vi "Write_Data.vi"(6 "Queues":T8, 8 "Status/Errors in":refnum<vi>, 9 "# Events to store":i32, 10 "Write data parameters in":T1 caption="Data Storage" {"Data storage"."Detector number" format="%#.0f"}) -> (0 "Status/Errors out":refnum<vi>, 2 "Write data parameters out":T1 {"Data storage"."Detector number" format="%#.0f"})   [LabVIEW 2013]
uses:
  Controls/Write_Data_Parameters.ctl
  Controls/Stop_Loop.ctl
  Controls/Data_Storage.ctl
  Controls/DB_Connection.ctl
  database/Connection.llb/Conn ObjectReference.ctl
  Controls/Data_Storage_Condition.ctl
  Controls/GPS_Timestamp.ctl
  Controls/Queues.ctl
  Controls/One_Second.ctl
  Controls/Get_Set_Statistics_Options2.ctl
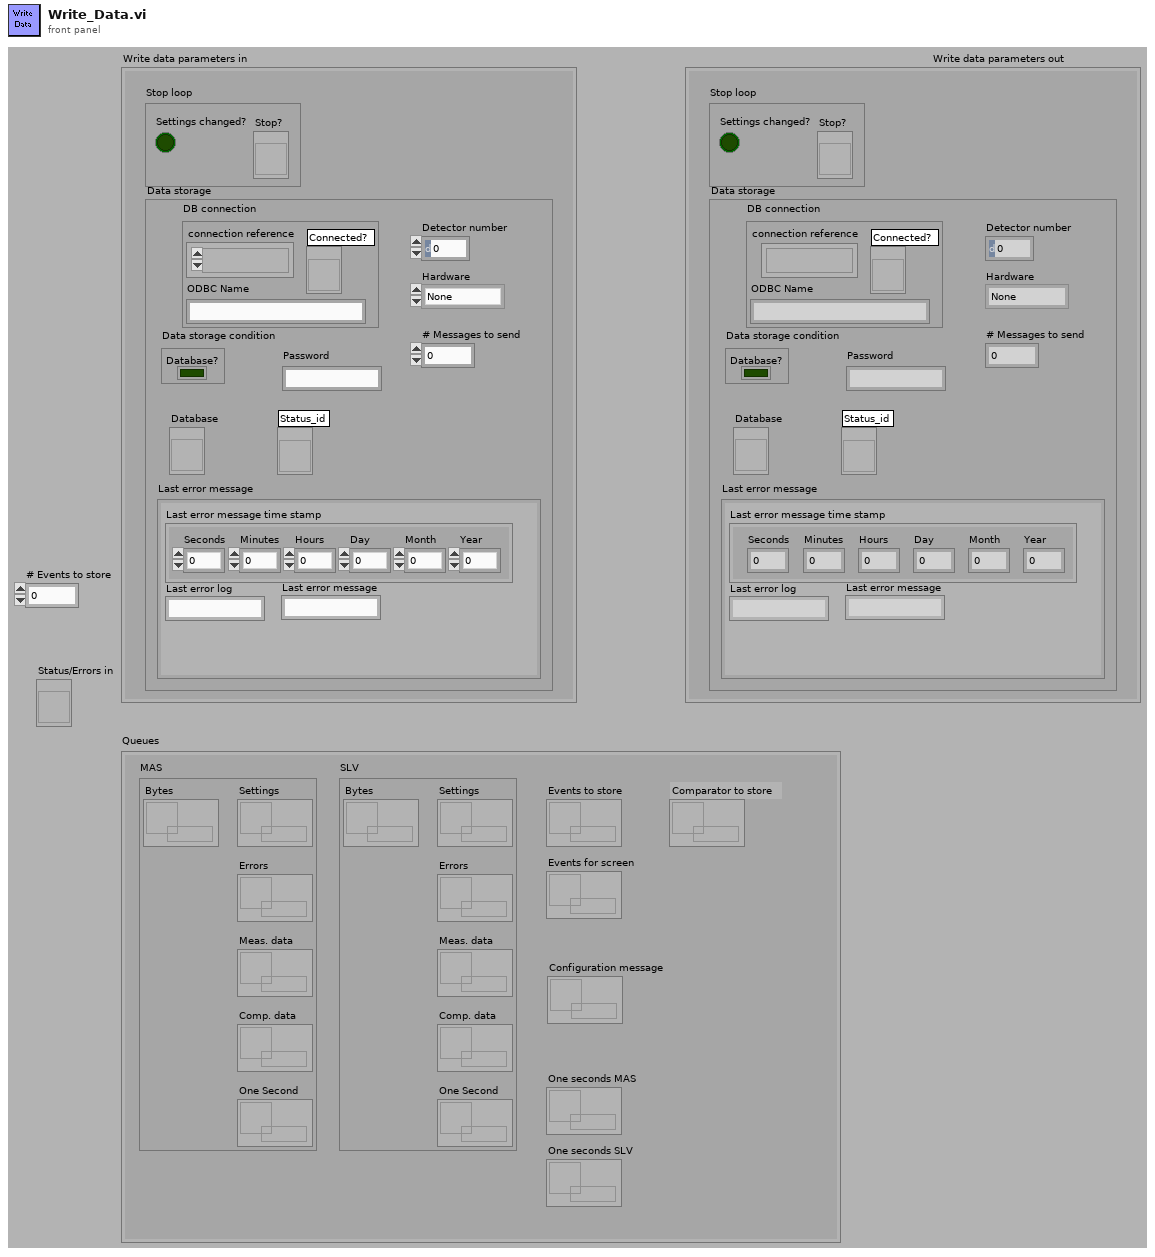
[diagram p1: front panel]
types:
  T1 = typedef "Write_Data_Parameters.ctl" = cluster{"Stop loop":T2, "Data storage":T3}
  T2 = typedef "Stop_Loop.ctl" = cluster{"Settings changed?":bool, "Stop?":refnum<vi>}
  T3 = typedef "Data_Storage.ctl" = cluster{"DB connection":T4, "Data storage condition":T6, "Detector number":u16, "# Messages to send":i32, "Database":refnum<vi>, "Password":string, "Last error message":cluster{"Last error message time stamp":T7, "Last error log":string, "Last error message":string}, "Status_id":refnum<vi>, "Hardware":enum8{"None", "HiSPARC I", "HiSPARC II", "HiSPARC III", "Unknown"}}
  T4 = typedef "DB_Connection.ctl" = cluster{"connection reference":T5, "Connected?":refnum<vi>, "ODBC Name":string}
  T5 = typedef "Conn ObjectReference.ctl" = refnum<k1>
  T6 = typedef "Data_Storage_Condition.ctl" = cluster{"Database?":bool}
  T7 = typedef "GPS_Timestamp.ctl" = cluster{"Seconds":u8, "Minutes":u8, "Hours":u8, "Day":u8, "Month":u8, "Year":u16}
  T8 = typedef "Queues.ctl" = cluster{"MAS":cluster{"Bytes":refnum<queue>, "Settings":refnum<queue>, "Errors":refnum<queue>, "Meas. data":refnum<queue>, "One Second":refnum<queue>, "Comp. data":refnum<queue>}, "SLV":cluster{"Bytes":refnum<queue>, "Settings":refnum<queue>, "Errors":refnum<queue>, "Meas. data":refnum<queue>, "One Second":refnum<queue>, "Comp. data":refnum<queue>}, "Events to store":refnum<queue>, "Events for screen":refnum<queue>, "One seconds MAS":refnum<queue>, "One seconds SLV":refnum<queue>, "Configuration message":refnum<queue>, "Comparator to store":refnum<queue>}
  T9 = typedef "Get_Set_Statistics_Options2.ctl" = enum16{"Get", "Set"}
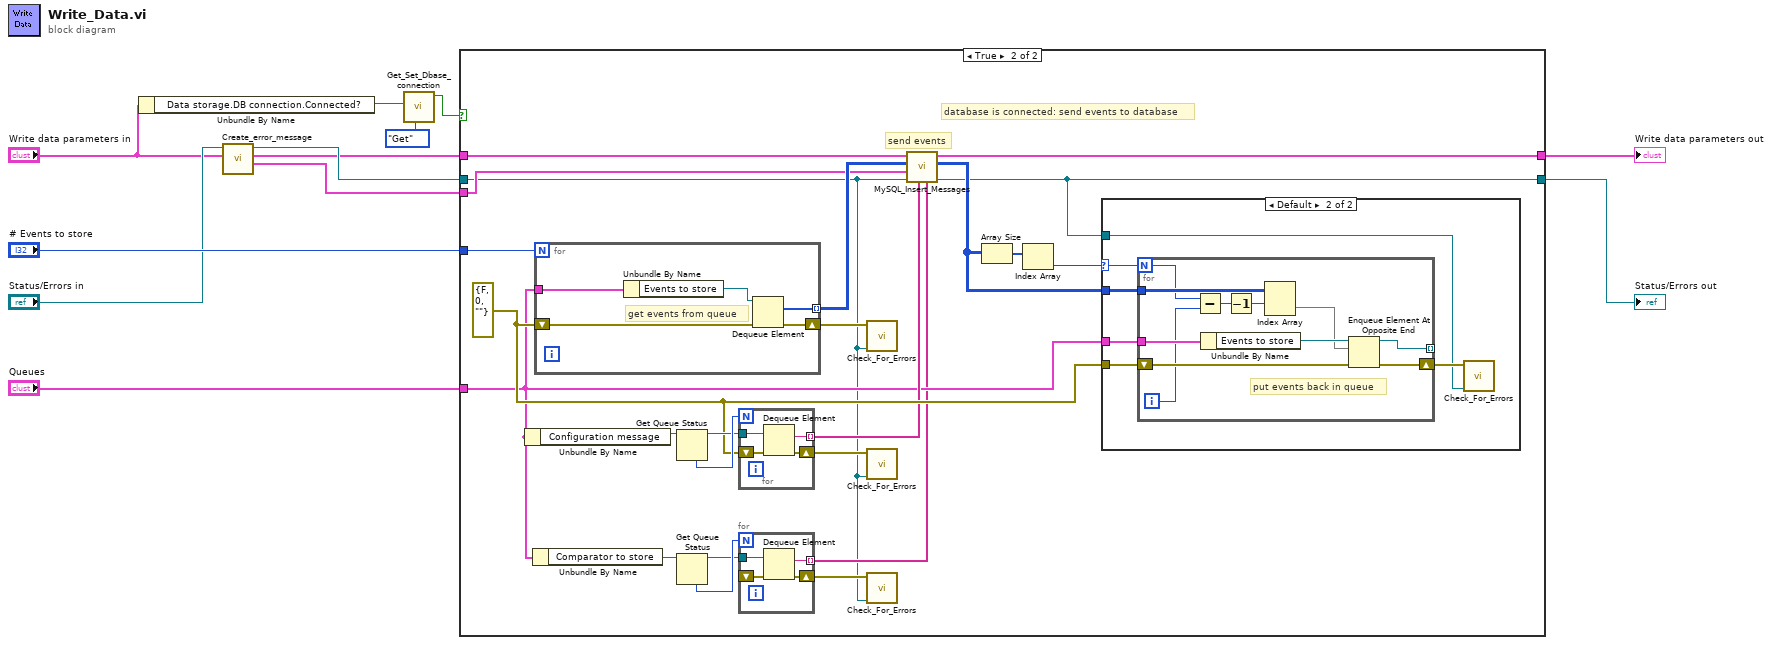
[diagram p0: block diagram]
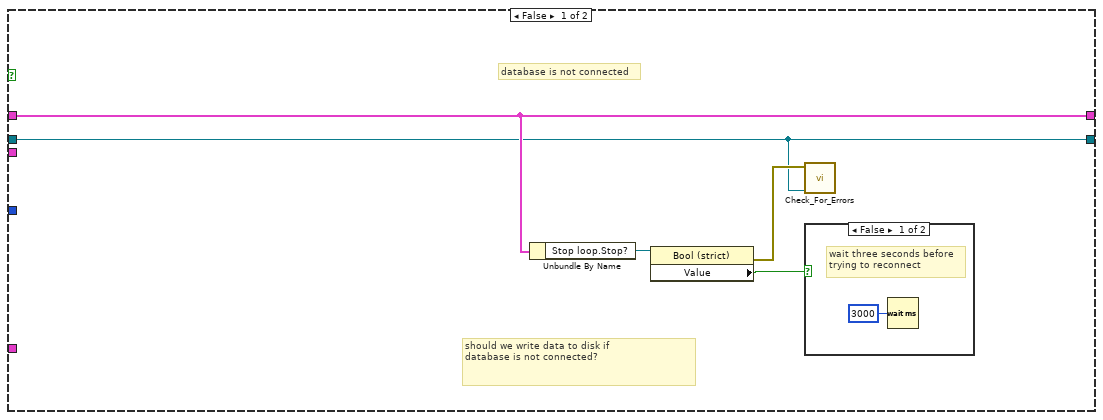
[diagram p2: hidden frame]
diagram:
  n1 = Unbundle By Name("Write data parameters in") -> ("Data storage.DB connection.Connected?"=w1:refnum<vi>)
  n2 = call "Create_error_message.vi"("Write data parameters in"="Write data parameters in", "Status/Errors in"="Status/Errors in") -> ("Error message"=w4:cluster{"New message ?":bool, "Message":string}, "Write data parameters out"=w5:T1, "Status/Errors out"=w7:refnum<vi>)  [unwired: 7 out]
  n3 = call "Get_Set_Dbase_connection.vi"("Get/Set"=Get_Set_Statistics_Options2."Get", "Connected? in"=w1) -> ("Value out"=w3:bool)  [unwired: 2 in, 7 out]
  n4 = case shown="True" w3 {
    tunnel: [w16 w41] -> w11
    tunnel: w5 -> [w16 w40]
    tunnel: "# Events to store" -> [_ w38]
    tunnel: w7 -> [w13 w19]
    tunnel: "Queues" -> [_ w21]
    tunnel: [w13 w34] -> w12
    tunnel: w4 -> [_ w32]
    frame False {
      # "should we write data to disk if\ndatabase is not connected?"
      # "database is not connected"
      n5 = Unbundle By Name(w16) -> ("Stop loop.Stop?"=w17:refnum<vi>)
      n6 = property class="Bool (strict)"(reference=w17) -> (error out=w14:errorcluster, "Value"=w15:bool)  [unwired: 1 in, 1 out]
      n7 = call "Check_For_Errors.vi"("Status/Errors in"=w13, "error in"=w14) -> ()  [unwired: 10 out]
      n8 = case shown="False" w15 {
        frame False {
          # "wait three seconds before\ntrying to reconnect"
          n9 = Wait (ms)(milliseconds to wait=u32 3000) -> ()  [unwired: 1 out]
        }
        frame True {
          # "don't wait and stop loop"
        }
      }
    }
    frame True {
      w28 = errorcluster {"status"=FALSE, "code"=0, "source"=""} ("error out")
      # "database is connected: send events to database"
      # "send events"
      n10 = Unbundle By Name(w21) -> ("Configuration message"=w31:refnum<queue>)
      n11 = Unbundle By Name(w21) -> ("Comparator to store"=w25:refnum<queue>)
      n12 = for {
        N: w38 -> [_]
        tunnel: [w70] -> w33 mode=indexing
        tunnel: w21 -> [w69]
        shift-right: [w67] -> w39
        shift-left: w28 -> [w68]
        # "get events from queue"
        n13 = Unbundle By Name(w69) -> ("Events to store"=w71:refnum<queue>)
        n14 = Dequeue Element(queue=w71, error in (no error)=w68) -> (element=w70:u8[], error out=w67:errorcluster)  [unwired: 3 out]
      }
      n15 = Get Queue Status(queue=w31) -> (queue out=w29:refnum<queue>, # elements in queue=w30:i32)  [unwired: 1 in, 7 out]
      n16 = Get Queue Status(queue=w25) -> (queue out=w23:refnum<queue>, # elements in queue=w24:i32)  [unwired: 1 in, 7 out]
      n17 = for {
        N: w30 -> [_]
        shift-right: [w47] -> w26
        shift-left: w28 -> [w48]
        tunnel: w29 -> [w49]
        tunnel: [w46] -> w27 mode=indexing
        n18 = Dequeue Element(queue=w49, error in (no error)=w48) -> (element=w46:string, error out=w47:errorcluster)  [unwired: 3 out]
      }
      n19 = for {
        N: w24 -> [_]
        shift-right: [w43] -> w22
        shift-left: _ -> [w44]
        tunnel: w23 -> [w45]
        tunnel: [w42] -> w20 mode=indexing
        n20 = Dequeue Element(queue=w45, error in (no error)=w44) -> (element=w42:string, error out=w43:errorcluster)  [unwired: 3 out]
      }
      n21 = call "Check_For_Errors.vi"("Status/Errors in"=w19, "error in"=w39) -> ()  [unwired: 10 out]
      n22 = call "Check_For_Errors.vi"("Status/Errors in"=w19, "error in"=w26) -> ()  [unwired: 10 out]
      n23 = call "Check_For_Errors.vi"("Status/Errors in"=w19, "error in"=w22) -> ()  [unwired: 10 out]
      n24 = call "MySQL_Insert_Messages.vi"("Comparator message"=w20, "Configuration messages"=w27, "Status/Errors in"=w19, "Error message"=w32, "Messages in"=w33, "Write data parameters in"=w40) -> ("Status/Errors out"=w34:refnum<vi>, "Messages out"=w35:u8[][], "Write data parameters out"=w41:T1)  [unwired: 3 out]
      n25 = Array Size(array=w35) -> (size(s)=w37:i32[])
      n26 = Index Array(array=w37) -> (element=w36:i32)  [unwired: 1 in]
      n27 = case shown="Default" w36 {
        selector: w36 -> [_ w53]
        tunnel: w21 -> [_ w54]
        tunnel: w35 -> [_ w52]
        tunnel: w34 -> [_ w51]
        tunnel: w28 -> [_ w50]
        frame 0 {
        }
        frame Default {
          n28 = for {
            N: w53 -> [w57]
            tunnel: [w64] -> _ mode=indexing
            tunnel: w54 -> [w63]
            shift-right: [w65] -> w55
            shift-left: w50 -> [w62]
            tunnel: w52 -> [w61]
            i -> [w56]
            # "put events back in queue"
            n29 = Subtract(x=w57, y=w56) -> (x-y=w58:i32)
            n30 = Unbundle By Name(w63) -> ("Events to store"=w66:refnum<queue>)
            n31 = Decrement(x=w58) -> (x-1=w60:i32)
            n32 = Index Array(array=w61, index (row)=w60) -> (element=w59:u8[])  [unwired: 1 in]
            n33 = Enqueue Element At Opposite End(queue=w66, element=w59, error in (no error)=w62) -> (queue out=w64:refnum<queue>, error out=w65:errorcluster)  [unwired: 2 out]
          }
          n34 = call "Check_For_Errors.vi"("Status/Errors in"=w51, "error in"=w55) -> ()  [unwired: 10 out]
        }
      }
    }
  }
  "Status/Errors out" <- w12
  "Write data parameters out" <- w11
